vi "Initialize Hardware References.vi"(8 "error in (no error)":errorcluster, 11 "Hardware Resources in":T1) -> (0 "error out":errorcluster, 3 "Hardware Resources out":T1)   [LabVIEW 2018, in "DAQ.lvlib" / "DAQ Write.lvlib"]
doc: "Initialize the hardware references."
uses:
  DAQ/DAQ Write.lvlib
  Hardware Configuration.ctl
  Acquisition/Task Cluster.ctl
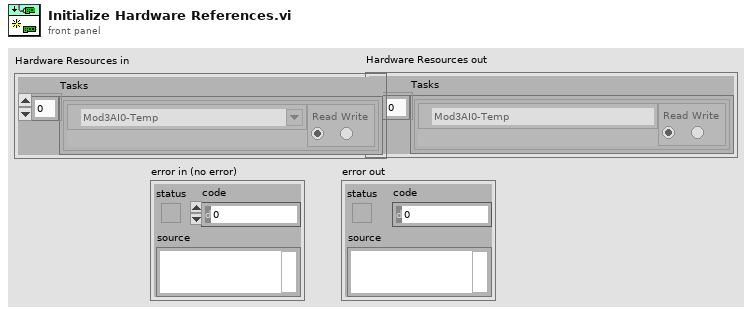
[diagram p1: front panel]
types:
  T1 = typedef "DAQ.lvlib/DAQ Write.lvlib/Hardware Configuration.ctl" = cluster{"Tasks":T2[]}
  T2 = typedef "Task Cluster.ctl" = cluster{"DAQmx Task":refnum<k21>, "Read-Write Radio":enum32{"Read", "Write"}}
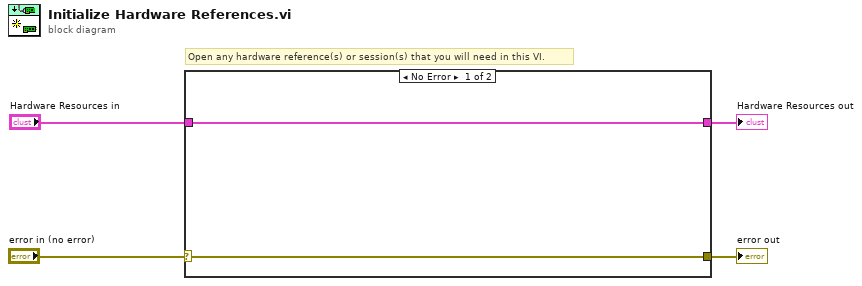
[diagram p0: block diagram]
diagram:
  # "Open any hardware reference(s) or session(s) that you will need in this VI."
  n1 = case shown="No Error" "error in (no error)" {
    selector: "error in (no error)" -> [w6 w7]
    tunnel: [w6 w7] -> w3
    tunnel: "Hardware Resources in" -> [w5 w8]
    tunnel: [w5 w8] -> w1
    frame No Error {
    }
    frame Error {
    }
  }
  "Hardware Resources out" <- w1
  "error out" <- w3
